vi "re_LuaVIEW Execute.vi"(5 "LuaVIEW reference in":T1, 11 "error in (no error)":errorcluster) -> (6 "LuaVIEW reference out":T1, 15 "error out":errorcluster)   [LabVIEW 2013]
doc: "Execute one or more previously compiled scripts until the last script completes or an error occurs and any cleanup handling has run its course. This simple iterator does not do run-time script management such as probing as tasks do. Neither does this VI allow for indexed functions to be called. To do that a custom iterator must be implemented."
uses:
  typedefs/t_LuaVIEW Reference.ctl
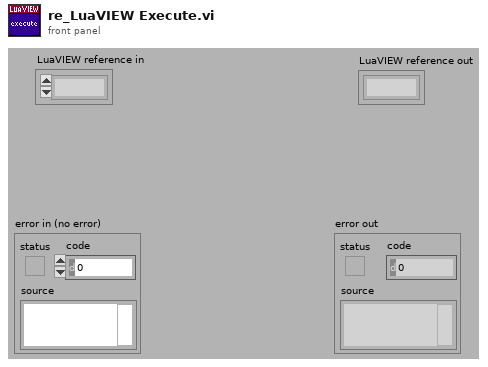
[diagram p1: front panel]
types:
  T1 = typedef "t_LuaVIEW Reference.ctl" = refnum<k1>
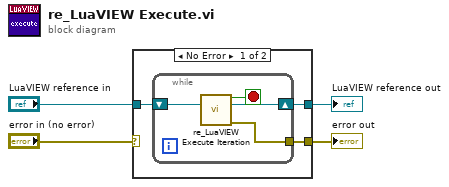
[diagram p0: block diagram]
diagram:
  n1 = case shown="No Error" "error in (no error)" {
    selector: "error in (no error)" -> [_ w13]
    tunnel: [w5 w13] -> w4
    tunnel: "LuaVIEW reference in" -> [w7 w12]
    tunnel: [w6 w12] -> w2
    frame No Error {
      n2 = while {
        shift-right: [w9] -> w6
        shift-left: w7 -> [w11]
        tunnel: [w8] -> w5
        stop <- w10 stop-if-true
        n3 = call "re_LuaVIEW Execute Iteration.vi"("LuaVIEW reference in"=w11) -> ("last?"=w10:bool, "LuaVIEW reference out"=w9:T1, "final error"=w8:errorcluster)  [unwired: 11 in, 1 out]
      }
    }
    frame Error {
    }
  }
  "error out" <- w4
  "LuaVIEW reference out" <- w2
